vi "Create and Read Recordset.vi"(5 "Max Rows to Fetch (-1 = all)":i32=-1, 6 "error in (no error)":errorcluster, 7 "Recordset Parameters":cluster{"CursorType":T1, "LockType":T2}={"CursorType"=0, "LockType"=1} {"LockType" items=["adLockUnspecified"=-1, "adLockReadOnly"=1, "adLockPessimistic"=2, "adLockOptimistic"=3, "adLockBatchOptimistic"=4]; "CursorType" items=["adOpenUnspecified"=-1, "adOpenForwardOnly"=0, "adOpenKeyset"=1, "adOpenDynamic"=2, "adOpenStatic"=3]}, 8 "Source":string, 9 "Connection In":refnum<k7>) -> (0 "error out":errorcluster, 1 "Rows Returned":i32, 2 "DB Data":string[][](table), 3 "Connection Out":refnum<k7>, 4 "Field Names Fetched":string[](array[string]))   [LabVIEW 2020, in "ADO Database Drivers.lvlib"]
uses:
  ADO Database Drivers.lvlib
  _typedefs/CursorType.ctl
  _typedefs/LockType.ctl
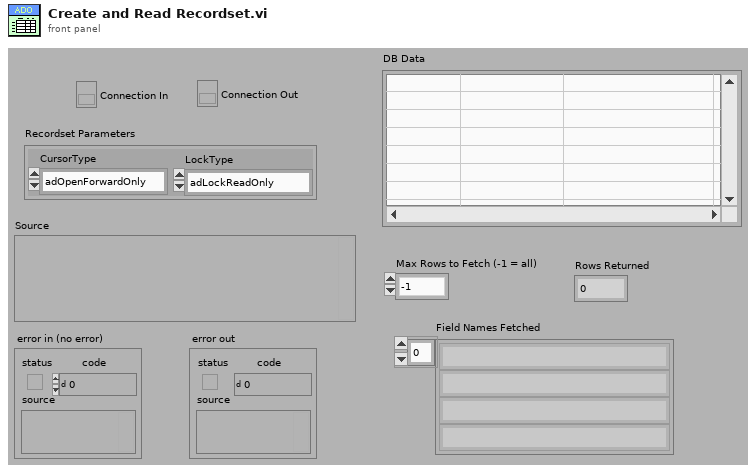
[diagram p1: front panel]
types:
  T1 = typedef "ADO Database Drivers.lvlib/CursorType.ctl" = i32
  T2 = typedef "ADO Database Drivers.lvlib/LockType.ctl" = i32
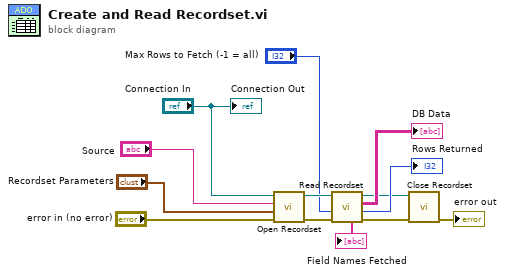
[diagram p0: block diagram]
diagram:
  n1 = call "Open Recordset.vi"("error in (no error)"="error in (no error)", "Recordset Parameters"="Recordset Parameters", "Source"="Source", "Connection"="Connection In") -> ("error out"=w13:errorcluster, "Recordset"=w12:refnum<k7>)  [unwired: 2 in]
  n2 = call "Read Recordset.vi"("Recordset In"=w12, "Max Rows to Fetch (-1 = all)"="Max Rows to Fetch (-1 = all)", "error in (no error)"=w13) -> ("Field Names"=→"Field Names Fetched":string[], "Recordset Out"=w5:refnum<k7>, "Data out"=→"DB Data":string[][], "Rows Returned"=→"Rows Returned":i32, "error out"=w11:errorcluster)  [unwired: 1 in]
  n3 = call "Close Recordset.vi"("error in"=w11, "Recordset"=w5) -> ("error out"=→"error out":errorcluster)  [unwired: 5 in]
  "Connection Out" <- "Connection In"
